vi "MicroBlaze_lwIP-Top.vi"() -> ()   [LabVIEW 2017, in "My Network Host v1.lvlib"]
uses:
  My Network Host v1.lvlib
  <vilib>/rvi/interface/nirviCloseFPGA/nirviCloseFPGA.xnode
  <vilib>/rvi/interface/nirviOpenFPGA/nirviOpenFPGA.xnode
  <vilib>/rvi/interface/nirviReadWriteControl/nirviReadWriteControl.xnode
  FPGA Bitfiles/0710GigabitCLIP_FPGATarget_Fpga-MicroBlazel_TxcRhwwxxSA.lvbitx
  FPGA/Fpga-MicroBlaze_lwIP.vi
  <vilib>/FPGAPlugInAG/PXIe-6592R/niLvFpga_Open_PXIe-6592R.vi
  <vilib>/rvi/interface/common/dynamic/niFpgaDynamicAddResources.vi
  NiFpgaLv.dll
  <vilib>/Utility/error.llb/Error Cluster From Error Code.vi
  <vilib>/rvi/interface/Simulation/niFpgaSimulationCallBeginRW.vi
  <vilib>/rvi/errors/niLvFpgaAdjustHostInterfaceError.vi
  <vilib>/FPGAPlugInAG/Dynamic/niLvFpga_Close_Dynamic.vi
  <vilib>/rvi/interface/nirviMethod/nirviMethod.xnode
  <vilib>/FPGAPlugInAG/Dynamic/niLvFpga_WriteFifo_Dynamic.vi
  <vilib>/rvi/errors/niLvFpgaMergeErrorWithErrorCode.vi
panel:
  in  "error in":errorcluster
  out "error out":errorcluster
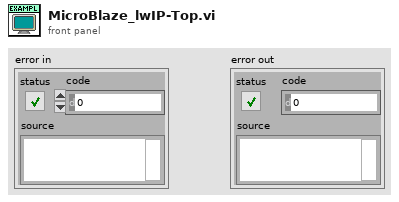
[diagram p1: front panel]
types:
  T1 = cluster{"mgtrefclks_valid":bool, "mgtrefclks_locked":bool, "posc_complete":bool, "sPort0_Power_Good":bool, "sPort1_Power_Good":bool, "signal_detect_Port0":bool, "signal_detect_Port1":bool}
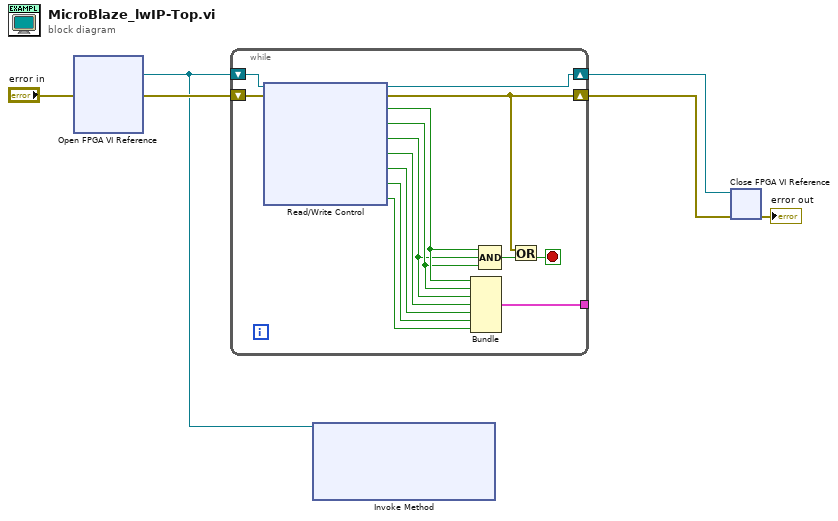
[diagram p0: block diagram]
diagram:
  n1 = xnode "Open FPGA VI Reference"("error in"="error in") -> ("FPGA VI Reference Out"=w1:refnum<k20>, "error out"=w5:errorcluster)  [unwired: 1 in]
  n2 = while {
    shift-right: [w19] -> w3
    shift-left: w1 -> [w20]
    shift-right: [w15] -> w2
    shift-left: w5 -> [w18]
    tunnel: [w7] -> _
    stop <- w16 stop-if-true
    n3 = xnode "Read/Write Control"("FPGA VI Reference In"=w20, "error in"=w18) -> ("FPGA VI Reference Out"=w19:refnum<k20>, "error out"=w15:errorcluster, "mgtrefclks_valid"=w14:bool, "mgtrefclks_locked"=w13:bool, "posc_complete"=w12:bool, "sPort0_Power_Good"=w11:bool, "sPort1_Power_Good"=w10:bool, "signal_detect_Port0"=w9:bool, "signal_detect_Port1"=w8:bool)
    n4 = Bundle("mgtrefclks_valid"=w14, "mgtrefclks_locked"=w13, "posc_complete"=w12, "sPort0_Power_Good"=w11, "sPort1_Power_Good"=w10, "signal_detect_Port0"=w9, "signal_detect_Port1"=w8) -> (w7:T1)  [unwired: 1 in]
    n5 = Compound Arithmetic op=AND(w14, w12, w13) -> (w17:bool)
    n6 = Or(x=w15, y=w17) -> (x .or. y?=w16:bool)
  }
  n7 = xnode "Invoke Method"("FPGA VI Reference In"=w1) -> ()  [unwired: 3 in, 3 out]
  n8 = xnode "Close FPGA VI Reference"("FPGA VI Reference In"=w3, "error in"=w2) -> ("error out"=→"error out":errorcluster)
